vi "QDInstrument_OptiCool_Example.vi"() -> ()   [LabVIEW 2021]
uses:
  <vilib>/Analysis/baseanly.llb/Mean (DBL).vi
  <vilib>/Analysis/NI_AALBase.lvlib
panel:
  in  "Remote":bool
  in  "IP Address":string="127.0.0.1"
  out "Field\nStatus":i32(ring) items=["MagnetUnknown"=0, "StablePersistent"=1, "WarmingSwitch"=2, "CoolingSwitch"=3, "StableDriven"=4, "Iterating"=5, "Charging"=6, "Discharging"=7, "CurrentError"=8, "MagnetFailure"=15]
  out "Temperature\nStatus":i32(ring) items=["TemperatureUnknown"=0, "Stable"=1, "Tracking"=2, "Near"=5, "Chasing"=6, "Filling"=7, "Standby"=10, "Disabled"=13, "ImpedanceNotFunction"=14, "TempFailure"=15]
  out "Field":dbl
  out "Measuring":bool
  in  "Delay":dbl=5.0
  in  "WaitForField":bool=TRUE
  in  "WaitForTemperature":bool=TRUE
  out "Temperature":dbl
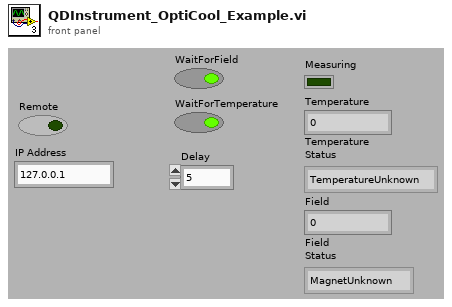
[diagram p1: front panel]
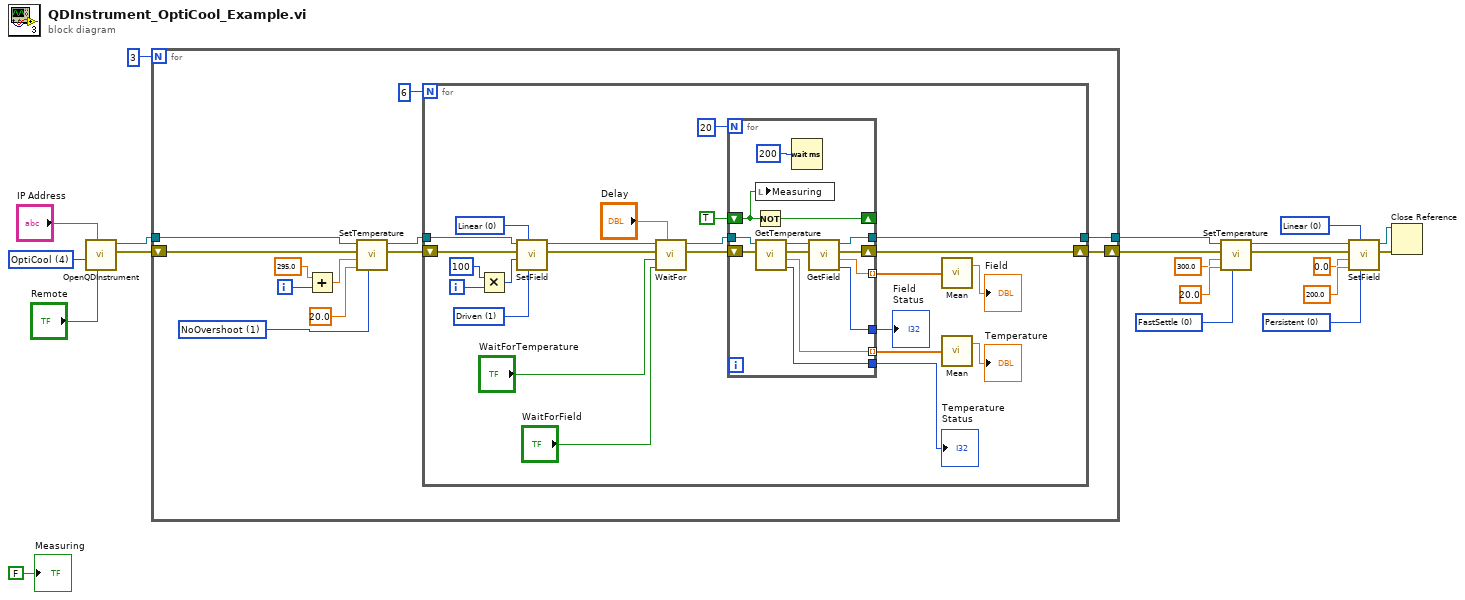
[diagram p0: block diagram]
diagram:
  w3 = 4 items=["PPMS", "VersaLab", "DynaCool", "SVSM", "OptiCool"] ("InstrumentType")
  w18 = 0 items=["Persistent", "Driven"] ("Mode")
  w17 = 0 items=["Linear", "NoOvershoot", "Oscillate"] ("Approach")
  w11 = 0 items=["FastSettle", "NoOvershoot"] ("Approach")
  n1 = call "OpenQDInstrument.vi"("Remote"="Remote", "IP Address"="IP Address", "InstrumentType"=w3) -> ("error out"=w1:errorcluster, "Instrument Ref"=w2:refnum<k24>)  [unwired: 5 in]
  n2 = for {
    N: 3 -> [_]
    shift-right: [w24] -> w10
    shift-left: w1 -> [w28]
    tunnel: w2 -> [w27]
    tunnel: [w21] -> w6
    i -> [w32]
    w22 = 1 items=["FastSettle", "NoOvershoot"] ("Approach")
    n3 = Add(x=295.0, y=w32) -> (x+y=w30:dbl)
    n4 = call "SetTemperature.vi"("Approach"=w22, "Rate"=20.0, "Temperature"=w30, "error in (no error)"=w28, "Instrument Ref In"=w27) -> ("error out"=w25:errorcluster, "Instrument Ref Out"=w26:refnum<k24>)  [unwired: 2 in, 1 out]
    n5 = for {
      N: 6 -> [_]
      tunnel: w26 -> [w49]
      shift-right: [w38] -> w24
      shift-left: w25 -> [w48]
      tunnel: [w41] -> w21
      i -> [w55]
      w53 = 0 items=["Linear", "NoOvershoot", "Oscillate"] ("Approach")
      w54 = 1 items=["Persistent", "Driven"] ("Mode")
      n6 = Multiply(x=100, y=w55) -> (x*y=w33:i32)
      n7 = call "SetField.vi"("Mode"=w54, "Approach"=w53, "Field"=w33, "error in (no error)"=w48, "Instrument Ref In"=w49) -> ("error out"=w47:errorcluster, "Instrument Ref Out"=w43:refnum<k24>)  [unwired: 2 in, 1 out]
      n8 = call "WaitFor.vi"("Delay"="Delay", "Wait For Field"="WaitForField", "Wait For Temperature"="WaitForTemperature", "error in (no error)"=w47, "Instrument Ref In"=w43) -> ("error out"=w52:errorcluster, "Instrument Ref Out"=w42:refnum<k24>)  [unwired: 5 in]
      n9 = for {
        N: 20 -> [_]
        shift-right: [w69] -> _
        shift-left: TRUE -> [w67]
        shift-right: [w64] -> w38
        shift-left: w52 -> [w66]
        tunnel: w42 -> [w63]
        tunnel: [w61] -> w41
        tunnel: [w58] -> w40
        tunnel: [w57] -> w39
        tunnel: [w59] -> w36 mode=indexing
        tunnel: [w60] -> w37 mode=indexing
        n10 = Not(x=w67) -> (.not. x?=w69:bool)
        n11 = local write "Measuring"(w67) -> ()
        n12 = call "GetTemperature.vi"("error in (no error)"=w66, "Instrument Ref In"=w63) -> ("Temperature\nStatus"=w57:i32, "Temperature"=w60:dbl, "error out"=w65:errorcluster, "Instrument Ref Out"=w62:refnum<k24>)  [unwired: 3 in, 1 out]
        n13 = Wait (ms)(milliseconds to wait=u32 200) -> ()  [unwired: 1 out]
        n14 = call "GetField.vi"("error in (no error)"=w65, "Instrument Ref In"=w62) -> ("Field\nStatus"=w58:i32, "Field"=w59:dbl, "error out"=w64:errorcluster, "Instrument Ref Out"=w61:refnum<k24>)  [unwired: 3 in, 1 out]
      }
      "Field\nStatus" <- w40
      "Temperature\nStatus" <- w39
      n15 = call-poly <vilib>:"Mean.vi"("X"=w36) -> ("mean"=→"Field":dbl)  [unwired: 1 out]
      n16 = call-poly <vilib>:"Mean.vi"("X"=w37) -> ("mean"=→"Temperature":dbl)  [unwired: 1 out]
    }
  }
  n17 = call "SetTemperature.vi"("Approach"=w11, "Rate"=20.0, "Temperature"=300.0, "error in (no error)"=w10, "Instrument Ref In"=w6) -> ("error out"=w14:errorcluster, "Instrument Ref Out"=w13:refnum<k24>)  [unwired: 2 in, 1 out]
  n18 = call "SetField.vi"("Mode"=w18, "Approach"=w17, "Rate"=200.0, "Field"=0.0, "error in (no error)"=w14, "Instrument Ref In"=w13) -> ("error out"=w20:errorcluster, "Instrument Ref Out"=w19:refnum<k24>)  [unwired: 1 in, 1 out]
  n19 = Close Reference(reference=w19, error in (no error)=w20) -> ()  [unwired: 1 out]
  "Measuring" <- FALSE
